vi "test High Priority Data - SA.vi"(8 "error in (no error)":errorcluster, 11 "BC Async SubRoutines in":refnum<class "BC Async SubRoutines.lvclass">) -> (0 "error out":errorcluster, 3 "BC Async SubRoutines out":refnum<class "BC Async SubRoutines.lvclass">)   [LabVIEW 2016, in "BC Async SubRoutines.lvclass"]
uses:
  BC Async SubRoutines.lvclass
  PPLs/FPGA Interface.lvlibp/FPGA Interface/FPGA Interface.lvclass
  Frames & Messages/Async Message/Async Message.lvclass
  Bus Controller/Bus Controller.lvclass
  1553 Component/1553 Component.lvclass
  Frames & Messages/TypeDefs/Message Control.ctl
  BCI-1553 API.lvlib
  Frames & Messages/TypeDefs/Command Config.ctl
  Frames & Messages/TypeDefs/Async Message Config.ctl
  Frames & Messages/TypeDefs/Command Word Count.ctl
  Frames & Messages/TypeDefs/Command SubAddress.ctl
  Frames & Messages/TypeDefs/Command Terminal Address.ctl
  Frames & Messages/TypeDefs/Command Type.ctl
  Dependencies/FPGA Interface/FPGA Interface.lvclass
panel:
  out "Data":u16[](array[numeric]) format="%04x"
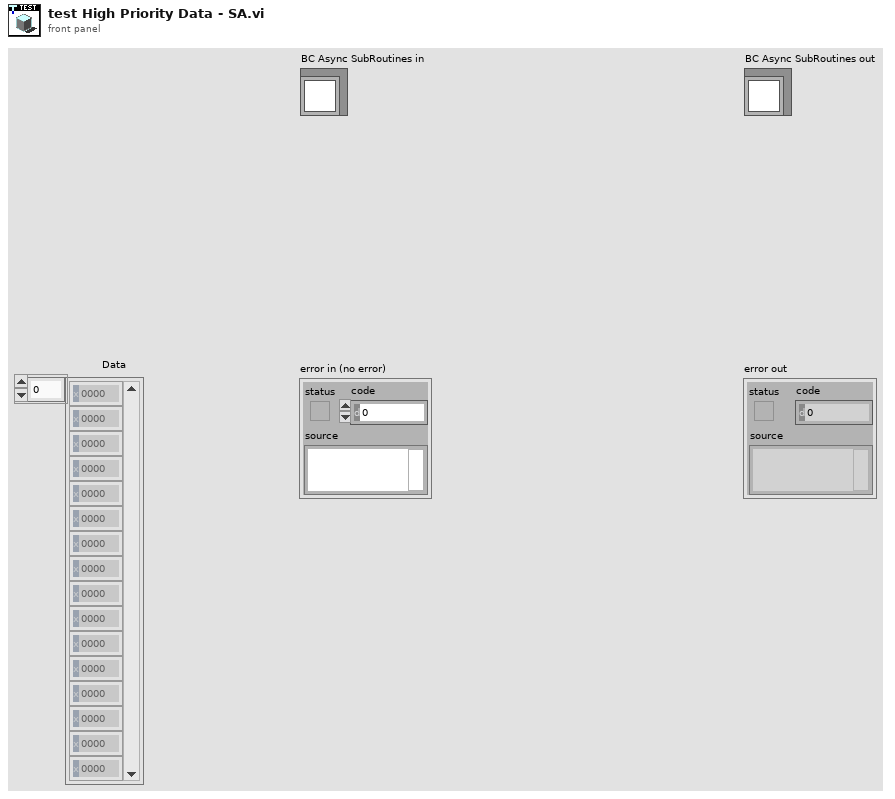
[diagram p1: front panel]
types:
  T1 = typedef "BCI-1553 API.lvlib/Command Config.ctl" = cluster{"Command Type":T2, "Terminal Address":T3, "SubAddress":T4, "Word Count\\Mode Code":T5, "Command Data":u16[]}
  T2 = typedef "BCI-1553 API.lvlib/Command Type.ctl" = enum16{"Transmit", "Receive"}
  T3 = typedef "BCI-1553 API.lvlib/Command Terminal Address.ctl" = enum16{"0", "1", "2", "3", "4", "5", "6", "7", "8", "9", "10", "11", "12", "13", "14", "15", "16", "17", "18", "19", "20", "21", "22", "23", "24", "25", "26", "27", "28", "29", "30", "Broadcast"}
  T4 = typedef "BCI-1553 API.lvlib/Command SubAddress.ctl" = enum16{"Mode Code", "1", "2", "3", "4", "5", "6", "7", "8", "9", "10", "11", "12", "13", "14", "15", "16", "17", "18", "19", "20", "21", "22", "23", "24", "25", "26", "27", "28", "29", "30"}
  T5 = typedef "BCI-1553 API.lvlib/Command Word Count.ctl" = enum16{"1", "2", "3", "4", "5", "6", "7", "8", "9", "10", "11", "12", "13", "14", "15", "16", "17", "18", "19", "20", "21", "22", "23", "24", "25", "26", "27", "28", "29", "30", "31", "32"}
  T6 = typedef "BCI-1553 API.lvlib/Async Message Config.ctl" = cluster{"Group":i32, "High Priority":bool, "Time to Next Msg (100 us)":u16, "Command Config":T1, "Message Control":T7}
  T7 = typedef "BCI-1553 API.lvlib/Message Control.ctl" = cluster{"MC17 Time Sync":bool, "Error Mask":bool, "Service Request Mask":bool, "Busy Mask":bool, "SubSystem Flag Mask":bool, "Terminal Flag Mask":bool, "Reserved Mask":bool, "Retry":bool, "Bus A / !Bus B":bool, "Self-Test Loopback":bool, "Broadcast Mask":bool, "EoM Interrupt":bool, "Mode Code Format":bool, "Broadcast Format":bool, "RT-RT Format":bool}
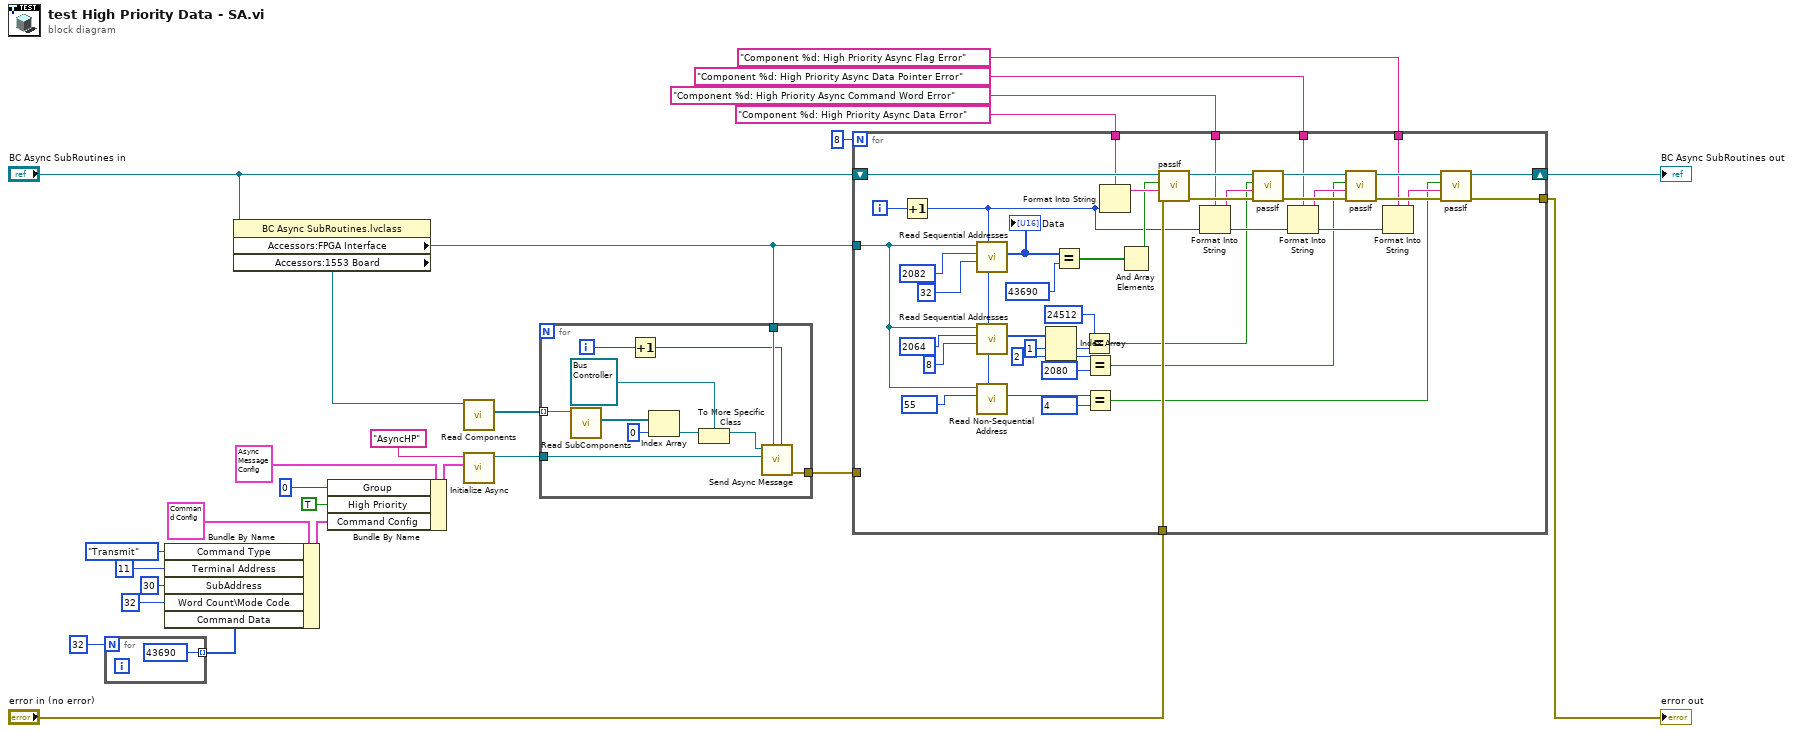
[diagram p0: block diagram]
diagram:
  n1 = for {
    N: 32 -> [_]
    tunnel: [u16 43690] -> w11 mode=indexing
  }
  n2 = Bundle By Name(cluster=T1 {"Command Type"=enum."Transmit", "Terminal Address"=enum."0", "SubAddress"=enum."Mode Code", "Word Count\\Mode Code"=enum."1", "Command Data"=[]} ("Command Config"), "Command Type"=enum16{"Transmit", "Receive"}."Transmit", "Terminal Address"=u16 11 ("Terminal Address (0-30)"), "SubAddress"=u16 30 ("SubAddress (1-30)"), "Word Count\\Mode Code"=u16 32 ("WC/MC (1-32)"), "Command Data"=w11) -> (w18:T1)
  n3 = property class="BC Async SubRoutines.lvclass"(reference="BC Async SubRoutines in") -> ("Accessors:FPGA Interface"=w9:refnum<class "FPGA Interface.lvclass">, "Accessors:1553 Board"=w24:refnum<class "1553 Board.lvclass">)  [unwired: 1 in, 2 out]
  n4 = Bundle By Name(cluster=T6 {"Group"=0, "High Priority"=FALSE, "Time to Next Msg (100 us)"=0, "Command Config"={"Command Type"=enum."Transmit", "Terminal Address"=enum."0", "SubAddress"=enum."Mode Code", "Word Count\\Mode Code"=enum."1", "Command Data"=[]}, "Message Control"={"MC17 Time Sync"=FALSE, "Error Mask"=FALSE, "Service Request Mask"=FALSE, "Busy Mask"=FALSE, "SubSystem Flag Mask"=FALSE, "Terminal Flag Mask"=FALSE, "Reserved Mask"=FALSE, "Retry"=FALSE, "Bus A / !Bus B"=FALSE, "Self-Test Loopback"=FALSE, "Broadcast Mask"=FALSE, "EoM Interrupt"=FALSE, "Mode Code Format"=FALSE, "Broadcast Format"=FALSE, "RT-RT Format"=FALSE}} ("Async Message Config"), "Group"=0, "High Priority"=TRUE, "Command Config"=w18) -> (w21:T6)
  n5 = call "Read Components.vi"("1553 Board in"=w24) -> ("Components"=w23:refnum<class "1553 Component.lvclass">[])  [unwired: 8 in, 2 out]
  n6 = call "Initialize Async.vi"("Async Message Config"=w21, "ID"="AsyncHP") -> ("Async Message out"=w10:refnum<class "Async Message.lvclass">)  [unwired: 8 in, 1 out]
  n7 = for {
    tunnel: w23 -> [w39] mode=indexing
    tunnel: w10 -> [w33]
    tunnel: w9 -> [w32]
    tunnel: [w29] -> w8
    i -> [w31]
    n8 = call "Read SubComponents.vi"("1553 Component in"=w39) -> ("SubComponents"=w38:refnum<class "1553 SubComponent.lvclass">[])  [unwired: 8 in, 2 out]
    n9 = Increment(x=w31) -> (x+1=w30:i32)
    n10 = Index Array(array=w38, index=0) -> (element=w36:refnum<class "1553 SubComponent.lvclass">)
    n11 = To More Specific Class(target class=refnum<class "Bus Controller.lvclass"> refnum ("SLSC 1553 API.lvlib:Bus Controller.lvclass"), reference=w36) -> (specific class reference=w34:refnum<class "Bus Controller.lvclass">)  [unwired: 1 in, 1 out]
    n12 = call-dynamic "Send Async Message.vi"("Component ID"=w30, "FPGA Interface"=w32, "Async Message"=w33, "Bus Controller in"=w34) -> ("error out"=w29:errorcluster)  [unwired: 6 in, 1 out]
  }
  n13 = for {
    N: 8 -> [_]
    tunnel: w9 -> [w62]
    shift-right: [w57] -> w3
    shift-left: "BC Async SubRoutines in" -> [w80]
    tunnel: "error in (no error)" -> [w79]
    tunnel: [w53] -> w2
    tunnel: "Component %d: High Priority Async Data Error" ("custom report message (\"\")") -> [w78]
    tunnel: w8 -> [_]
    tunnel: "Component %d: High Priority Async Command Word Error" ("custom report message (\"\")") -> [w52]
    tunnel: "Component %d: High Priority Async Data Pointer Error" ("custom report message (\"\")") -> [w51]
    tunnel: "Component %d: High Priority Async Flag Error" ("custom report message (\"\")") -> [w50]
    i -> [w81]
    n14 = Increment(x=w81) -> (x+1=w46:i32)
    n15 = call-dynamic "Read Sequential Addresses.vi"("Target IC (1-8)"=w46, "Addresses to Read"=u16 32, "Starting Address"=u16 2082, "FPGA Interface in"=w62) -> ("Data"=w71:u16[])  [unwired: 6 in, 1 out]
    "Data" <- w71
    n16 = call-dynamic "Read Sequential Addresses.vi"("Target IC (1-8)"=w46, "Addresses to Read"=u16 8, "Starting Address"=u16 2064, "FPGA Interface in"=w62) -> ("Data"=w68:u16[])  [unwired: 6 in, 1 out]
    n17 = call-dynamic "Read Non-Sequential Address.vi"("Target IC (1-8)"=w46, "Address"=u16 55, "FPGA Interface in"=w62) -> ("Data"=w40:u16)  [unwired: 7 in, 1 out]
    n18 = Index Array(array=w68, index #1=1 ("index"), index #2=2 ("index")) -> (element #1=w64:u16, element #2=w41:u16)
    n19 = Equal?(x=w71, y=u16 43690) -> (x = y?=w69:bool[])
    n20 = Equal?(x=u16 24512, y=w64) -> (x = y?=w45:bool)
    n21 = Equal?(x=w41, y=u16 2080) -> (x = y?=w44:bool)
    n22 = Equal?(x=w40, y=u16 4) -> (x = y?=w43:bool)
    n23 = Format Into String(format string=w78, w46) -> (resulting string=w77:string)  [unwired: 2 in, 1 out]
    n24 = And Array Elements(Boolean array=w69) -> (logical AND=w75:bool)
    n25 = call-dynamic "passIf.vi"("error in (no error)"=w79, "message (\"\")"=w77, "pass"=w75, "TestCase in"=w80) -> ("error out"=w56:errorcluster, "TestCase out"=w58:refnum<class "BC Async SubRoutines.lvclass">)  [unwired: 6 in]
    n26 = Format Into String(format string=w52, w46) -> (resulting string=w47:string)  [unwired: 2 in, 1 out]
    n27 = call-dynamic "passIf.vi"("error in (no error)"=w56, "message (\"\")"=w47, "pass"=w45, "TestCase in"=w58) -> ("error out"=w55:errorcluster, "TestCase out"=w60:refnum<class "BC Async SubRoutines.lvclass">)  [unwired: 6 in]
    n28 = Format Into String(format string=w51, w46) -> (resulting string=w48:string)  [unwired: 2 in, 1 out]
    n29 = call-dynamic "passIf.vi"("error in (no error)"=w55, "message (\"\")"=w48, "pass"=w44, "TestCase in"=w60) -> ("error out"=w54:errorcluster, "TestCase out"=w59:refnum<class "BC Async SubRoutines.lvclass">)  [unwired: 6 in]
    n30 = Format Into String(format string=w50, w46) -> (resulting string=w49:string)  [unwired: 2 in, 1 out]
    n31 = call-dynamic "passIf.vi"("error in (no error)"=w54, "message (\"\")"=w49, "pass"=w43, "TestCase in"=w59) -> ("error out"=w53:errorcluster, "TestCase out"=w57:refnum<class "BC Async SubRoutines.lvclass">)  [unwired: 6 in]
  }
  "error out" <- w2
  "BC Async SubRoutines out" <- w3
